vi "Stop Core.vi"(10 "final error code":i32, 11 "Classic Logger in":refnum<class "Classic Logger.lvclass">) -> (3 "Classic Logger out":refnum<class "Classic Logger.lvclass">)   [LabVIEW 2017, in "MGI-Monitored Actor.lvlib" / "Classic Logger.lvclass"]
doc: "(<B>Filename</B>: Actor Framework.lvlib:Actor.lvclass:Stop Core.vi)\n\nDefines what the actor does before it stops. Use the <B>final error code</B> input to determine whether the actor shut down in response to an error.\n\nBy default, this method does nothing. A descendant class may override it to define behavior, such as shutting down any processes the actor initiated in its override of the Actor Core method."
uses:
  Classic Logger.lvclass
  Classic Logger.lvclass/Classic Logger.ctl
  <vilib>/ActorFramework/Actor/Actor.lvclass
  monitored-actor-core/Source/Monitored Actor/Monitored Actor Messages/Disable Message Logging Msg/Disable Message Logging Msg.lvclass
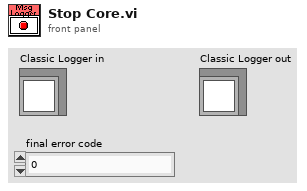
[diagram p1: front panel]
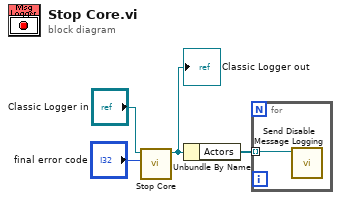
[diagram p0: block diagram]
diagram:
  n1 = call-parent "Stop Core.vi"("final error code"="final error code", "Actor in"="Classic Logger in") -> ("Actor out"=w2:refnum<class "Classic Logger.lvclass">)  [unwired: 9 in]
  "Classic Logger out" <- w2
  n2 = Unbundle By Name(w2) -> ("Actors"=w1:refnum<class "Message Enqueuer.lvclass">[])
  n3 = for {
    tunnel: w1 -> [w5] mode=indexing
    n4 = call "Send Disable Message Logging.vi"("Message Enqueuer in"=w5) -> ()  [unwired: 9 in, 2 out]
  }
